vi "Close_Devices_Main_v1.vi"(8 "error in":errorcluster, 11 "Resources in":T1 {"ZI ModHandle"."ModHandle" format="0x%08x"; "ZI ModHandle"."Conn" format="0x%08x"; "ZI Handle"."Handle" format="0x%08x"; "ZI Handle"."Conn" format="0x%08x"}) -> (0 "error out":errorcluster)   [LabVIEW 2021]
uses:
  Resources.ctl
  <instrlib>/Zurich Instruments LabOne/Public/ziTypeHandle.ctl
  <instrlib>/Zurich Instruments LabOne/Public/Modules/ziTypeModHandle.ctl
  <instrlib>/Zurich Instruments LabOne/Zurich Instruments LabOne.lvlib
  <instrlib>/Keithley 622x LV 2009/Keithley 622x.lvlib
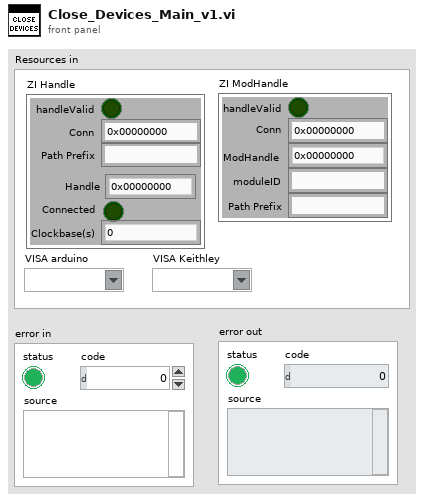
[diagram p1: front panel]
types:
  T1 = typedef "Resources.ctl" = cluster{"ZI Handle":T2, "ZI ModHandle":T3, "VISA arduino":refnum<visa-resource-name>, "VISA Keithley":refnum<visa-resource-name>}
  T2 = typedef "Zurich Instruments LabOne.lvlib/ziTypeHandle.ctl" = cluster{"handleValid":bool, "Conn":u64, "Path Prefix":string, "Handle":u64, "Connected":bool, "Clockbase(s)":dbl}
  T3 = typedef "Zurich Instruments LabOne.lvlib/ziTypeModHandle.ctl" = cluster{"handleValid":bool, "Conn":u64, "ModHandle":u64, "moduleID":string, "Path Prefix":string}
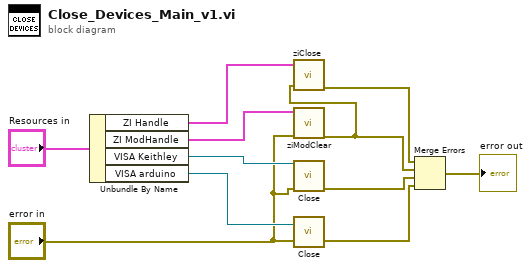
[diagram p0: block diagram]
diagram:
  n1 = Unbundle By Name("Resources in") -> ("ZI Handle"=w7:T2, "ZI ModHandle"=w8:T3, "VISA Keithley"=w9:refnum<visa-resource-name>, "VISA arduino"=w10:refnum<visa-resource-name>)
  n2 = call <instrlib>:"ziModClear.vi"("Error In"="error in", "ziModHandle In"=w8) -> ("Error Out"=w1:errorcluster)  [unwired: 7 in, 1 out]
  n3 = call <instrlib>:"ziClose.vi"("Error In"=w1, "Handle In"=w7) -> ("Error Out"=w5:errorcluster)  [unwired: 2 in, 1 out]
  n4 = call <instrlib>:"Close.vi"("VISA resource name"=w9, "error in (no error)"="error in") -> ("error out"=w4:errorcluster)  [unwired: 13 in]
  n5 = call <instrlib>:"Close.vi"("error in"="error in", "VISA arduino in"=w10) -> ("error out"=w3:errorcluster)  [unwired: 1 in]
  n6 = Merge Errors(w5, w1, w4, w3) -> (→"error out":errorcluster)
